vi "FTW-Reflection-VIServer.vi"(7 "VI Server Reference":variant) -> (6 "Data Name":string, 8 "Class Name":string, 10 "Class ID":u32, 14 "Payload Size":i16 format="%d bytes")   [LabVIEW 2015]
panel:
  # "Inputs"
  # "Outputs"
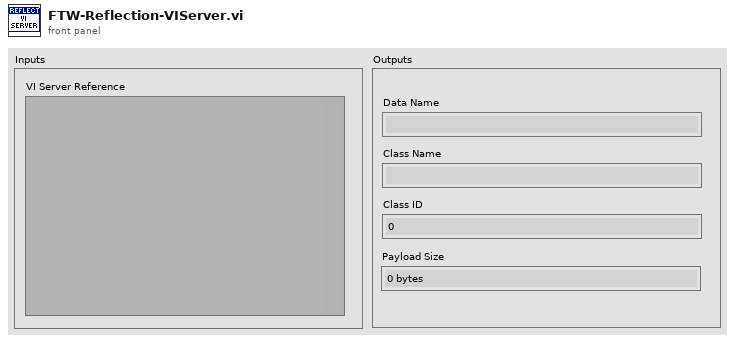
[diagram p1: front panel]
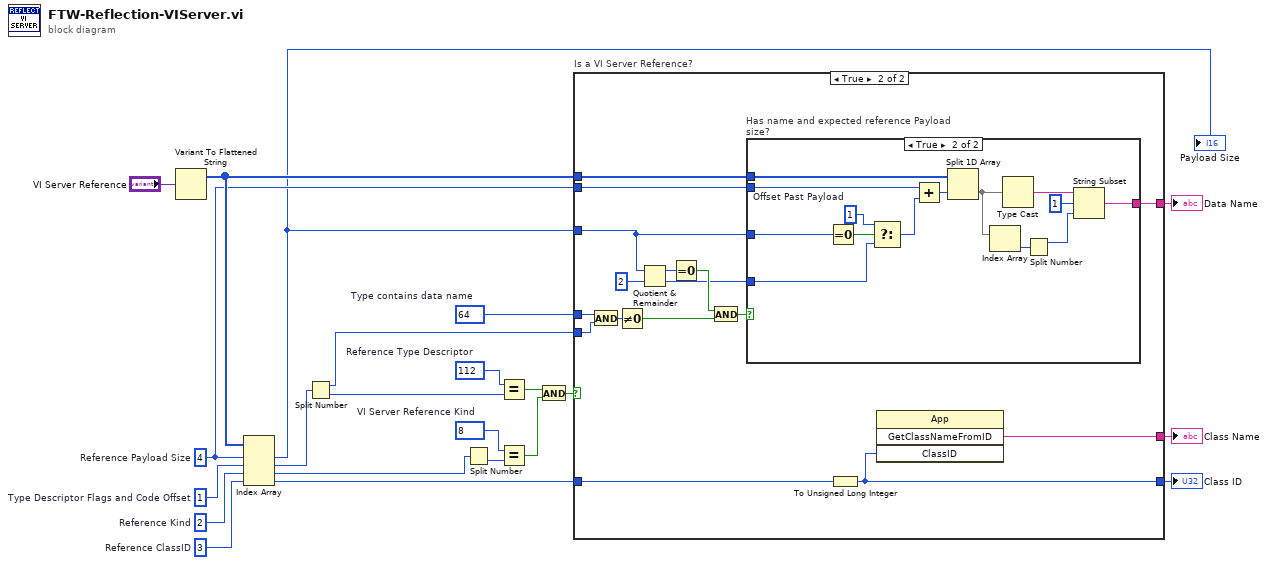
[diagram p0: block diagram]
diagram:
  w3 = 4  # Reference Payload Size
  w5 = u8 64  # Type contains data name
  w10 = u8 8  # VI Server Reference Kind
  w14 = u8 112  # Reference Type Descriptor
  w16 = 3  # Reference ClassID
  w17 = 2  # Reference Kind
  w22 = 1  # Type Descriptor Flags and Code Offset
  n1 = Variant To Flattened String(Variant="VI Server Reference") -> (1:w4:i16[])  [unwired: 1 out]
  n2 = Index Array(array=w4, index #1=w3, index #2=w22, index #3=w17, index #4=w16) -> (element #1=w1:i16, element #2=w21:i16, element #3=w12:i16, element #4=w15:i16)
  "Payload Size" <- w1
  n3 = Split Number(x=w21) -> (hi(x)=w6:u8, lo(x)=w13:u8)
  n4 = Split Number(x=w12) -> (lo(x)=w11:u8)  [unwired: 1 out]
  n5 = Equal?(x=w14, y=w13) -> (x = y?=w8:bool)
  n6 = Equal?(x=w10, y=w11) -> (x = y?=w9:bool)
  n7 = And(x=w8, y=w9) -> (x .and. y?=w7:bool)
  n8 = case "Is a VI Server Reference?" shown="True" w7 {
    tunnel: [_ w38] -> w19
    tunnel: [_ w36] -> w18
    tunnel: w15 -> [_ w37]
    tunnel: w6 -> [_ w34]
    tunnel: w5 -> [_ w35]
    tunnel: w1 -> [_ w24]
    tunnel: w4 -> [_ w23]
    tunnel: w3 -> [_ w30]
    tunnel: [_ w25] -> w2
    frame False {
    }
    frame True {
      n9 = And(x=w35, y=w34) -> (x .and. y?=w33:u8)
      n10 = Not Equal To 0?(x=w33) -> (x != 0?=w28:bool)
      n11 = Quotient & Remainder(x=w24, y=i16 2) -> (x-y*floor(x/y)=w31:i16, floor(x/y)=w26:i16)
      n12 = Equal To 0?(x=w31) -> (x = 0?=w29:bool)
      n13 = And(x=w29, y=w28) -> (x .and. y?=w27:bool)
      n14 = case "Has name and expected reference Payload size?" shown="True" w27 {
        tunnel: w23 -> [_ w52]
        tunnel: w24 -> [_ w50]
        tunnel: w30 -> [_ w48]
        tunnel: w26 -> [_ w45]
        tunnel: [_ w42] -> w25
        frame False {
        }
        frame True {
          w46 = 1  # Offset Past Payload
          n15 = Equal To 0?(x=w50) -> (x = 0?=w51:bool)
          n16 = Select(t=w46, s=w51, f=w45) -> (s? t:f=w49:i32)
          n17 = Add(x=w48, y=w49) -> (x+y=w47:i32)
          n18 = Split 1D Array(array=w52, index=w47) -> (second subarray=w41:i16[])  [unwired: 1 out]
          n19 = Index Array(array=w41) -> (element=w40:i16)  [unwired: 1 in]
          n20 = Type Cast(x=w41) -> (*(type *) &x=w44:string)  [unwired: 1 in]
          n21 = Split Number(x=w40) -> (hi(x)=w39:u8)  [unwired: 1 out]
          n22 = String Subset(string=w44, offset (0)=1 ("length (rest)"), length (rest)=w39) -> (substring=w42:string)
        }
      }
      n23 = To Unsigned Long Integer(number=w37) -> (unsigned 32bit integer=w36:u32)
      n24 = invoke class="App" method="GetClassNameFromID"("ClassID"=w36) -> ("GetClassNameFromID"=w38:string)  [unwired: 3 in, 3 out]
    }
  }
  "Data Name" <- w2
  "Class Name" <- w19
  "Class ID" <- w18
